vi "helper_move_motor.vi"(8 "Move step size":i32, 11 "input cluster":T2) -> (2 "output cluster":T1)   [LabVIEW 2014]
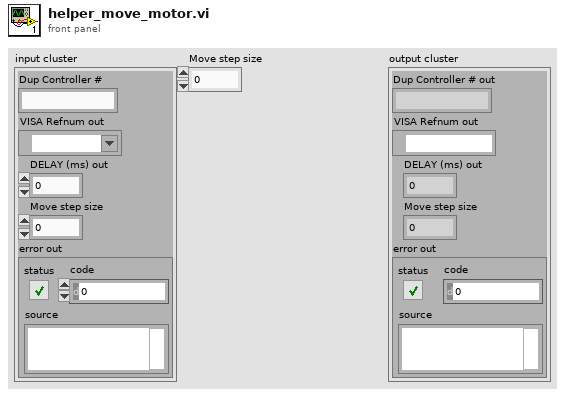
[diagram p1: front panel]
types:
  T1 = cluster{"Dup Controller # out":string, "VISA Refnum out":refnum<visa-resource-name>, "DELAY (ms) out":u32, "Move step size":i32, "error out":errorcluster}
  T2 = cluster{"Dup Controller #":string, "VISA Refnum out":refnum<visa-resource-name>, "DELAY (ms) out":u32, "Move step size":i32, "error out":errorcluster}
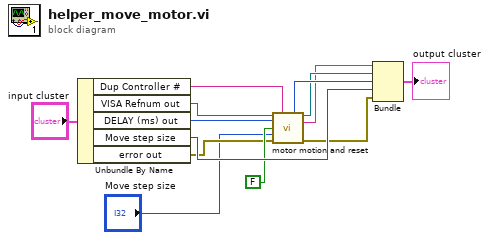
[diagram p0: block diagram]
diagram:
  n1 = Unbundle By Name("input cluster") -> ("Dup Controller #"=w4:string, "VISA Refnum out"=w5:refnum<visa-resource-name>, "DELAY (ms) out"=w6:u32, "Move step size"=w13:i32, "error out"=w7:errorcluster)
  n2 = call "motor motion and reset.vi"("VISA Refnum in"=w5, "Dup Controller # in"=w4, "DELAY (ms) in"=w6, "Reset"=FALSE, "Move step size"="Move step size", "error in (no error)"=w7) -> ("DELAY (ms) out"=w11:u32, "VISA Refnum out"=w10:refnum<visa-resource-name>, "Dup Controller # out"=w9:string, "error out"=w12:errorcluster)  [unwired: 4 in, 2 out]
  n3 = Bundle("Dup Controller # out"=w9, "VISA Refnum out"=w10, "DELAY (ms) out"=w11, "Move step size"=w13, "error out"=w12) -> (→"output cluster":T1)  [unwired: 1 in]
